vi "emi_Is Time Elapsed.vi"(5 "Start Time(ms)":u32, 7 "Timeout":u32, 9 "error in (no error)":errorcluster) -> (6 "Time Elapsed(ms)":u32, 8 "Time Elapsed?":bool, 10 "error out":errorcluster)   [LabVIEW 2010]
doc: "Used to see if a certain number of ms has elapsed, must be called to check. Can be used for having polling loops timeout.\n\nHas no internal memory, so starttime must be input at all times.\n\nOn Error in. No change in behavior"
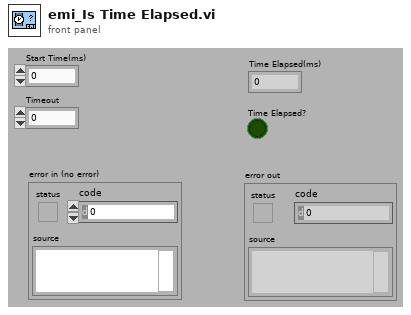
[diagram p1: front panel]
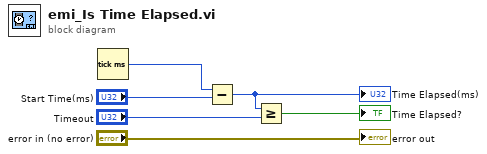
[diagram p0: block diagram]
diagram:
  n1 = Tick Count (ms)() -> (millisecond timer value=w6:u32)
  n2 = Subtract(x=w6, y="Start Time(ms)") -> (x-y=w2:u32)
  "Time Elapsed(ms)" <- w2
  n3 = Greater Or Equal?(x=w2, y="Timeout") -> (x >= y?=→"Time Elapsed?":bool)
  "error out" <- "error in (no error)"
